vi "Xsens LatLon (SubVI).vi"(5 "DATA in (Hex)":string) -> (0 "Channel Units":string[](array[string])=["NA", "YYYY", "MM", "dd", "hh", "mm", "ss", "NA", "ns", "NA", "NA", "NA", "NA", "DD", "DD", "mm", "mm", "mm", "mm"], 1 "Channel DataTypes":string[](array[string])=["Double Float", "Double Float"], 2 "Lat/Lon":string[](array[string]), 3 "Channel Names":string[](array[string]))   [LabVIEW 2019]
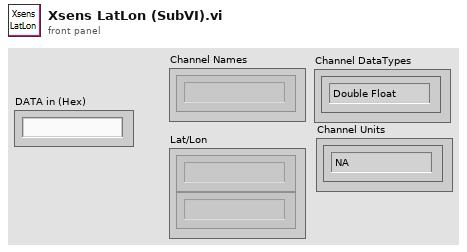
[diagram p1: front panel]
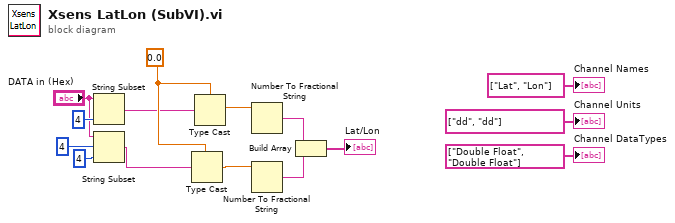
[diagram p0: block diagram]
diagram:
  w15 = sgl 0.0
  n1 = String Subset(string="DATA in (Hex)", length (rest)=4 ("length (rest)")) -> (substring=w13:string)  [unwired: 1 in]
  n2 = String Subset(string="DATA in (Hex)", offset (0)=4, length (rest)=4 ("length (rest)")) -> (substring=w10:string)
  n3 = Type Cast(type=w15, x=w10) -> (*(type *) &x=w6:sgl)
  n4 = Type Cast(type=w15, x=w13) -> (*(type *) &x=w8:sgl)
  n5 = Number To Fractional String(number=w8) -> (F-format string=w7:string)  [unwired: 3 in]
  n6 = Number To Fractional String(number=w6) -> (F-format string=w5:string)  [unwired: 3 in]
  n7 = Build Array(w7, w5) -> (→"Lat/Lon":string[])
  "Channel Names" <- string[] ["Lat", "Lon"] ("Channel Names")
  "Channel Units" <- string[] ["dd", "dd"]
  "Channel DataTypes" <- string[] ["Double Float", "Double Float"]
